vi "PCDeviceInit.vi"(10 "error in (no error)":errorcluster) -> ()   [LabVIEW 2011]
uses:
  Utilities/controls/ctlSeqFNs_Main.ctl
  Utilities/controls/ctlSeqFNs_AVTGuppy.ctl
  Utilities/controls/ctlSeqFNs_CTIOTF.ctl
  Utilities/controls/ctlSeqFNs_Koheras.ctl
  Utilities/controls/ctlSeqFNs_PCDeviceInit.ctl
  Utilities/controls/ctlSeqFNs_Scanner.ctl
  Utilities/controls/ctlSeqFNs_Andor.ctl
  <vilib>/userDefined/High Color/IMAQdx.ctl
panel:
  in  "config remote device":T2
  in  "initDevData":T3
  in  "StatusTerminal":string[](array[string])
  in  "remote device online status":T4
  in  "interface management remote device":T5
  in  "set remote device online":T4
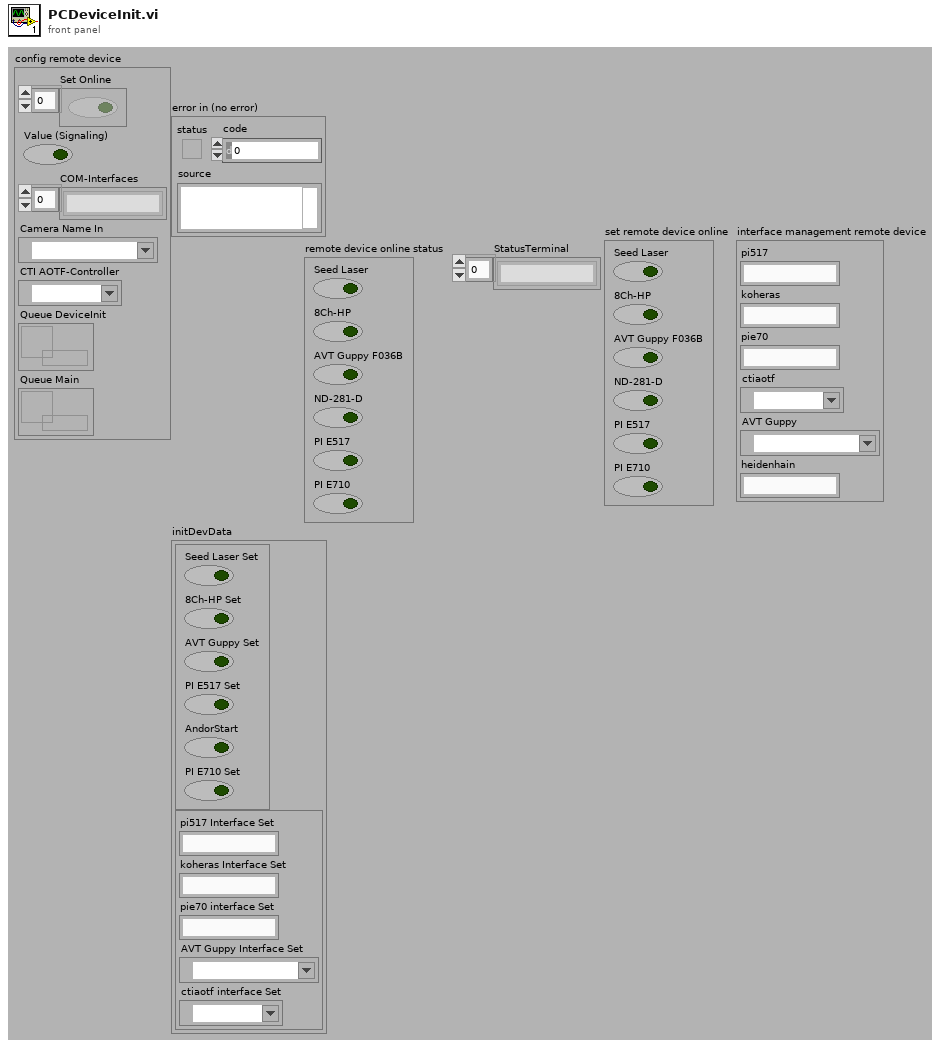
[diagram p1: front panel]
types:
  T1 = typedef "IMAQdx.ctl" = refnum<k21>
  T2 = cluster{"Set Online":bool[], "Value (Signaling)":bool, "COM-Interfaces":string[], "Camera Name In":T1, "CTI AOTF-Controller":refnum<visa-resource-name>, "Queue DeviceInit":refnum<queue>, "Queue Main":refnum<queue>}
  T3 = cluster{cluster{"Seed Laser Set":bool, "8Ch-HP Set":bool, "AVT Guppy Set":bool, "PI E517 Set":bool, "AndorStart":bool, "PI E710 Set":bool}, cluster{"pi517 Interface Set":string, "koheras Interface Set":string, "pie70 interface Set":string, "AVT Guppy Interface Set":T1, "ctiaotf interface Set":refnum<visa-resource-name>}}
  T4 = cluster{"Seed Laser":bool, "8Ch-HP":bool, "AVT Guppy F036B":bool, "ND-281-D":bool, "PI E517":bool, "PI E710":bool}
  T5 = cluster{"pi517":string, "koheras":string, "pie70":string, "ctiaotf":refnum<visa-resource-name>, "AVT Guppy":T1, "heidenhain":string}
  T6 = typedef "ctlSeqFNs_PCDeviceInit.ctl" = enum16{"ERROR", "INIT", "ErrorDevice", "StartDevice", "DeviceStatus", "StopDevice", "EXIT", "IDLE"}
  T7 = cluster{"Queue Main":refnum<queue>, "Queue Andor":refnum<queue>, "Queue Scanner":refnum<queue>, "Queue Koheras":refnum<queue>, "Queue CTIOTF":refnum<queue>, "Queue AVTGuppy":refnum<queue>, "set remote device online":cluster{"Seed Laser":bool, "8Ch-HP":bool, "AVT Guppy F036B":bool, "ND-281-D":bool, "PI E517":bool, "PI E710":bool}, "config remote device":cluster{"Set Online":bool[], "Value (Signaling)":bool, "COM-Interfaces":string[], "Camera Name In":T1, "CTI AOTF-Controller":refnum<visa-resource-name>, "Queue DeviceInit":refnum<queue>, "Queue Main":refnum<queue>}, "remote device online status":cluster{"Seed Laser":bool, "8Ch-HP":bool, "AVT Guppy F036B":bool, "ND-281-D":bool, "PI E517":bool, "PI E710":bool}, "interface management remote device":cluster{"pi517":string, "koheras":string, "pie70":string, "ctiaotf":refnum<visa-resource-name>, "AVT Guppy":T1, "heidenhain":string}, "StatusTerminal":string[], "initDevData":cluster{cluster{"Seed Laser Set":bool, "8Ch-HP Set":bool, "AVT Guppy Set":bool, "PI E517 Set":bool, "AndorStart":bool, "PI E710 Set":bool}, cluster{"pi517 Interface Set":string, "koheras Interface Set":string, "pie70 interface Set":string, "AVT Guppy Interface Set":T1, "ctiaotf interface Set":refnum<visa-resource-name>}}}
  T8 = typedef "ctlSeqFNs_Koheras.ctl" = enum16{"ERROR", "INIT", "Initialization", "Configuration", "Measurement", "Shutdown", "IDLE", "EXIT"}
  T9 = typedef "ctlSeqFNs_Andor.ctl" = enum16{"ERROR", "INIT", "Initialization", "Configuration", "Measurement", "Shutdown", "IDLE", "EXIT"}
  T10 = typedef "ctlSeqFNs_Scanner.ctl" = enum16{"ERROR", "INIT", "Initialization", "Configuration", "Measurement", "Shutdown", "IDLE", "EXIT"}
  T11 = typedef "ctlSeqFNs_CTIOTF.ctl" = enum16{"ERROR", "INIT", "Initialization", "Configuration", "Measurement", "Shutdown", "IDLE", "EXIT"}
  T12 = typedef "ctlSeqFNs_AVTGuppy.ctl" = enum16{"ERROR", "INIT", "Initialization", "Configuration", "Measurement", "Shutdown", "IDLE", "EXIT"}
  T13 = typedef "ctlSeqFNs_Main.ctl" = enum16{"ERROR", "INIT", "CONFIGURE", "MEASUREMENT", "SHUTDOWN", "IDLE", "EXIT"}
  T14 = cluster{"pi517 Interface Set":string, "pie70 interface Set":string, "PI E710":bool, "PI E517":bool}
  T15 = cluster{"Koheras":bool, "AOTF":bool, "ctiaotf interface Set":refnum<visa-resource-name>, "koheras Interface Set":string}
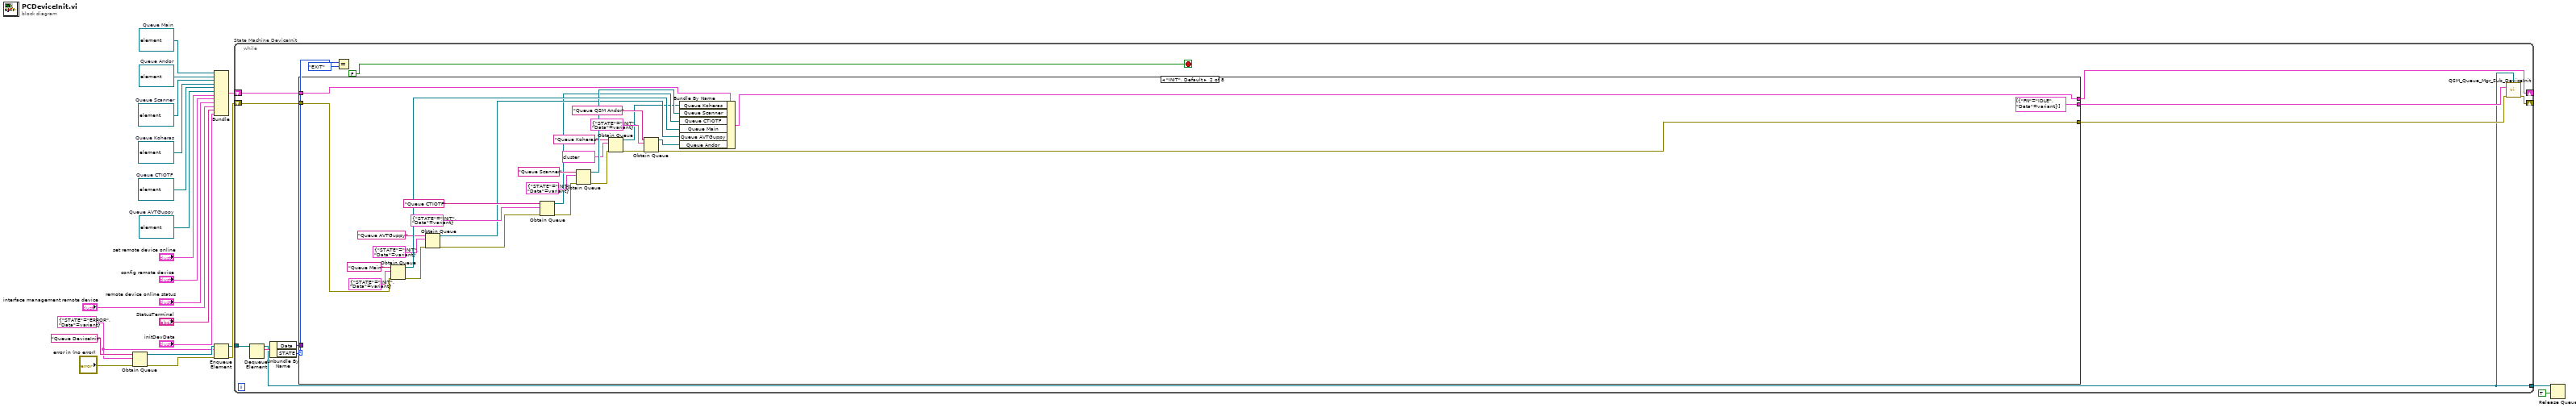
[diagram p0: block diagram]
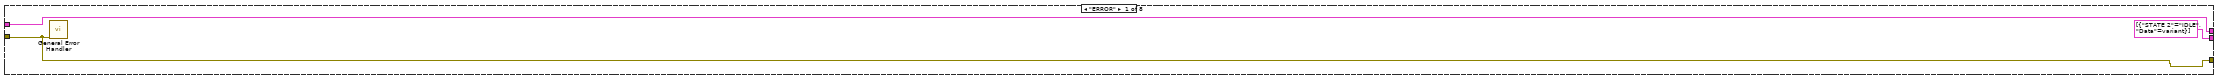
[diagram p2: hidden frame]
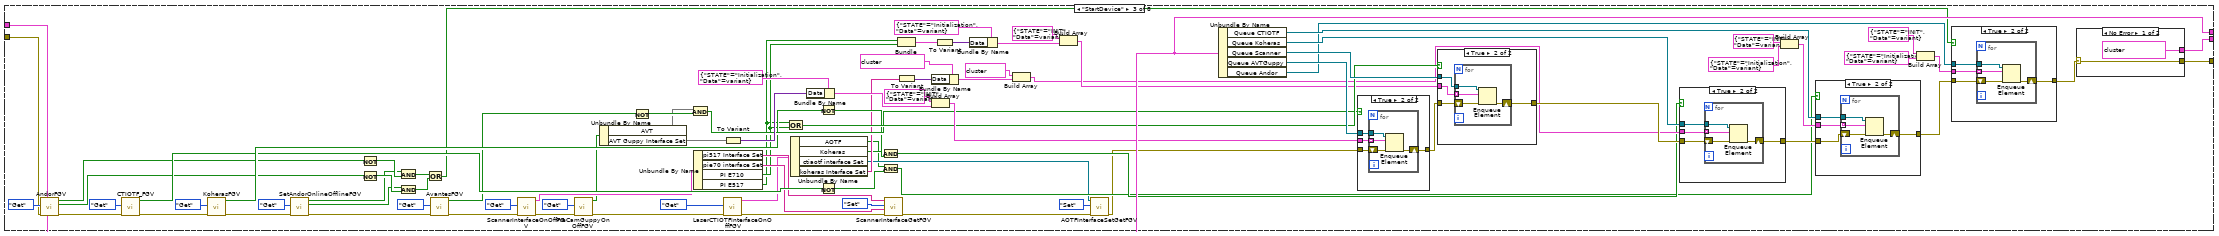
[diagram p3: hidden frame]
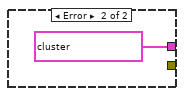
[diagram p9: hidden frame]
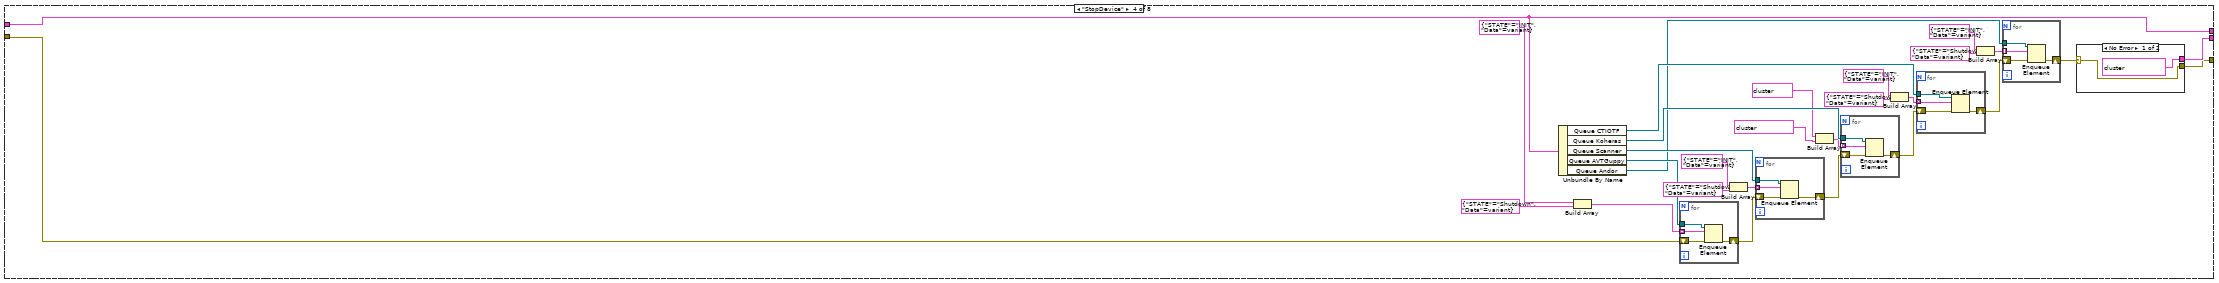
[diagram p10: hidden frame]
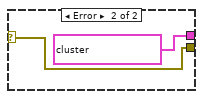
[diagram p11: hidden frame]
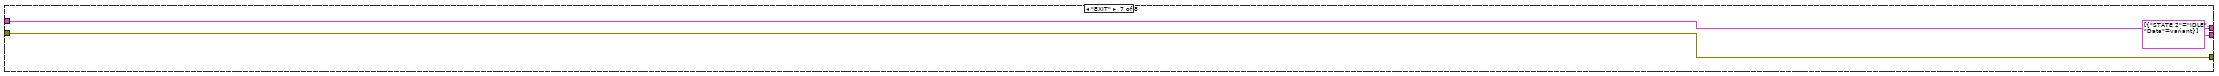
[diagram p14: hidden frame]
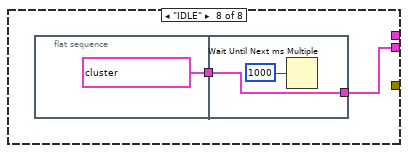
[diagram p15: hidden frame]
diagram:
  w1 = refnum<queue> refnum  # Queue Koheras
  w5 = refnum<queue> refnum  # Queue Andor
  w6 = refnum<queue> refnum  # Queue CTIOTF
  w7 = refnum<queue> refnum  # Queue AVTGuppy
  w9 = refnum<queue> refnum  # Queue Scanner
  w4 = refnum<queue> refnum  # Queue Main
  w14 = cluster{"STATE":T6, "Data":variant} {"STATE"=enum."ERROR", "Data"=variant} ("element")
  n1 = Obtain Queue(name (unnamed)="Queue DeviceInit", element data type=w14, error in (no error)="error in (no error)") -> (queue out=w19:refnum<queue>, error out=w21:errorcluster)  [unwired: 2 in, 1 out]
  n2 = Bundle("Queue Main"=w4, "Queue Andor"=w5, "Queue Scanner"=w9, "Queue Koheras"=w1, "Queue CTIOTF"=w6, "Queue AVTGuppy"=w7, "set remote device online"="set remote device online", "config remote device"="config remote device", "remote device online status"="remote device online status", "interface management remote device"="interface management remote device", "StatusTerminal"="StatusTerminal", "initDevData"="initDevData") -> (w18:T7)  [unwired: 1 in]
  n3 = Enqueue Element(queue=w19, element=w14, error in (no error)=w21) -> (queue out=w15:refnum<queue>, error out=w20:errorcluster)  [unwired: 1 in, 1 out]
  n4 = while "State Machine DeviceInit" {
    shift-right: [w28] -> _
    shift-left: w20 -> [w35]
    tunnel: w15 -> [w34]
    tunnel: [w26] -> w17
    shift-right: [w30] -> _
    shift-left: w18 -> [w31]
    stop <- FALSE ("x = y?") stop-if-true
    n5 = Dequeue Element(queue=w34) -> (queue out=w26:refnum<queue>, element=w33:cluster{"STATE":T6, "Data":variant})  [unwired: 2 in, 2 out]
    n6 = Unbundle By Name(w33) -> ("Data"=w32:variant, "STATE"=w25:T6)
    n7 = case shown="\"INIT\", Default" w25 {
      tunnel: w35 -> [w36 w65 w91 w205 w256 _ w260 _]
      tunnel: w32 -> [_ _ _ _ _ _ _ _]
      tunnel: w31 -> [w38 w66 w154 w206 w257 _ w259 _]
      tunnel: [w38 w48 w154 w206 w257 _ w259 _] -> w30
      tunnel: [cluster{"STATE 2":T6, "Data":variant}[] [{"STATE 2"=enum."IDLE", "Data"=variant}] cluster{"FN":T6, "Data":variant}[] [{"FN"=enum."IDLE", "Data"=variant}] w150 w231 _ _ cluster{"STATE 2":T6, "Data":variant}[] [{"STATE 2"=enum."IDLE", "Data"=variant}] w261] -> w27
      tunnel: [w36 w44 w149 w230 w256 _ w260 _] -> w29
      frame "ERROR" {
        n8 = call <vilib>:"General Error Handler.vi"("error in (no error)"=w36) -> ()  [unwired: 10 in, 5 out]
      }
      frame "INIT", Default {
        n9 = Obtain Queue(name (unnamed)="Queue Main" ("Queue Name"), element data type=cluster{"STATE":T13, "Data":variant} {"STATE"=enum."INIT", "Data"=variant} ("element"), error in (no error)=w65) -> (queue out=w62:refnum<queue>, error out=w60:errorcluster)  [unwired: 2 in, 1 out]
        n10 = Obtain Queue(name (unnamed)="Queue AVTGuppy" ("Queue Name"), element data type=cluster{"STATE":T12, "Data":variant} {"STATE"=enum."INIT", "Data"=variant} ("element"), error in (no error)=w60) -> (queue out=w51:refnum<queue>, error out=w55:errorcluster)  [unwired: 2 in, 1 out]
        n11 = Obtain Queue(name (unnamed)="Queue CTIOTF", element data type=cluster{"STATE":T11, "Data":variant} {"STATE"=enum."INIT", "Data"=variant} ("element"), error in (no error)=w55) -> (queue out=w47:refnum<queue>, error out=w52:errorcluster)  [unwired: 2 in, 1 out]
        n12 = Obtain Queue(name (unnamed)="Queue Scanner", element data type=cluster{"STATE":T10, "Data":variant} {"STATE"=enum."INIT", "Data"=variant} ("element"), error in (no error)=w52) -> (queue out=w54:refnum<queue>, error out=w53:errorcluster)  [unwired: 2 in, 1 out]
        n13 = Obtain Queue(name (unnamed)="Queue Koheras", element data type=cluster{"Data":variant, "FGV_Control":T8} {"Data"=variant, "FGV_Control"=enum."INIT"} ("element"), error in (no error)=w53) -> (queue out=w39:refnum<queue>, error out=w45:errorcluster)  [unwired: 2 in, 1 out]
        n14 = Obtain Queue(name (unnamed)="Queue QSM Andor", element data type=cluster{"STATE":T9, "Data":variant} {"STATE"=enum."INIT", "Data"=variant} ("element"), error in (no error)=w45) -> (queue out=w43:refnum<queue>, error out=w44:errorcluster)  [unwired: 2 in, 1 out]
        n15 = Bundle By Name(cluster=w66, "Queue Koheras"=w39, "Queue Scanner"=w54, "Queue CTIOTF"=w47, "Queue Main"=w62, "Queue AVTGuppy"=w51, "Queue Andor"=w43) -> (w48:T7)
      }
      frame "StartDevice" {
        n16 = call "AndorFGV.vi"("error in"=w91, "Set_Get"=enum16{"Set", "Get"}."Get") -> ("error out"=w90:errorcluster, "andor 1"=w100:bool, "andor 0"=w110:bool)  [unwired: 7 in]
        n17 = call "CTIOTF_FGV.vi"("error in"=w90, "Set_Get"=enum16{"Set", "Get"}."Get") -> ("error out"=w89:errorcluster, "aotfGet"=w112:bool)  [unwired: 8 in]
        n18 = call "KoherasFGV.vi"("error in"=w89, "Set_Get"=enum16{"Set", "Get"}."Get") -> ("error out"=w71:errorcluster, "Get"=w114:bool)  [unwired: 8 in]
        n19 = call "SetAndorOnlineOfflineFGV.vi"("error in"=w71, "Set_Get"=enum16{"Set", "Get"}."Get") -> ("error out"=w70:errorcluster, "andor 1"=w67:bool, "andor 0"=w68:bool)  [unwired: 7 in]
        n20 = Not(x=w110) -> (.not. x?=w109:bool)
        n21 = Not(x=w100) -> (.not. x?=w101:bool)
        n22 = And(x=w68, y=w109) -> (x .and. y?=w98:bool)
        n23 = And(x=w67, y=w101) -> (x .and. y?=w97:bool)
        n24 = Or(x=w98, y=w97) -> (x .or. y?=w99:bool)
        n25 = call "AvantesFGV.vi"("error in"=w70, "Set_Get"=enum16{"Set", "Get"}."Get") -> ("error out"=w88:errorcluster, "Get"=w108:bool)  [unwired: 8 in]
        n26 = call "ScannerInterfaceOnOffFGV.vi"("error in"=w88, "Set_Get"=enum16{"Set", "Get"}."Get") -> ("error out"=w94:errorcluster, "ScannerInterfaceOUT"=w84:T14)  [unwired: 8 in]
        n27 = call "PreCamGuppyOnOffFGV.vi"("error in"=w94, "Set_Get"=enum16{"Set", "Get"}."Get") -> ("error out"=w93:errorcluster, "out"=w79:bool)  [unwired: 8 in]
        n28 = Unbundle By Name(w79) -> ("AVT"=w77, "AVT Guppy Interface Set"=w78)
        n29 = Not(x=w108) -> (.not. x?=w107:bool)
        n30 = And(x=w77, y=w107) -> (x .and. y?=w120:bool)
        n31 = Unbundle By Name(w84) -> ("pi517 Interface Set"=w83:string, "pie70 interface Set"=w82:string, "PI E710"=w81:bool, "PI E517"=w80:bool)
        n32 = call "LaserCTIOTFInterfaceOnOffFGV.vi"("error in"=w93, "Set_Get"=enum16{"Set", "Get"}."Get") -> ("error out"=w92:errorcluster, "LaserCtiotfInterfaceOnOffOUT"=w76:T15)  [unwired: 8 in]
        n33 = To Variant(anything=w78) -> (Variant=w152:variant)
        n34 = Or(x=w80, y=w81) -> (x .or. y?=w142:bool)
        n35 = Unbundle By Name(w76) -> ("AOTF"=w72:bool, "Koheras"=w73:bool, "ctiaotf interface Set"=w74:refnum<visa-resource-name>, "koheras Interface Set"=w75:string)
        n36 = Bundle By Name(cluster=cluster{"STATE":T12, "Data":variant} {"STATE"=enum."Initialization", "Data"=variant} ("element"), "Data"=w152) -> (w148:cluster{"STATE":T12, "Data":variant})
        n37 = Not(x=w114) -> (.not. x?=w113:bool)
        n38 = Not(x=w112) -> (.not. x?=w111:bool)
        n39 = And(x=w73, y=w113) -> (x .and. y?=w124:bool)
        n40 = And(x=w72, y=w111) -> (x .and. y?=w122:bool)
        n41 = call "ScannerInterfaceGetFGV.vi"("error in"=w92, "pie70 interface Set"=w82, "FGV_Control"=enum16{"Set", "Get"}."Set", "pi517 Interface Set"=w83) -> ("error out"=w103:errorcluster)  [unwired: 5 in, 2 out]
        n42 = Bundle("PI E517"=w80, "PI E710"=w81) -> (w115:cluster{"PI E517":bool, "PI E710":bool})  [unwired: 1 in]
        n43 = To Variant(anything=w75) -> (Variant=w151:variant)
        n44 = Bundle By Name(cluster=cluster{"Data":variant, "FGV_Control":T8} {"Data"=variant, "FGV_Control"=enum."Initialization"} ("element"), "Data"=w151) -> (w137:cluster{"Data":variant, "FGV_Control":T8})
        n45 = Build Array(cluster{"STATE":T12, "Data":variant} {"STATE"=enum."INIT", "Data"=variant} ("element"), w148) -> (w146:cluster{"STATE":T12, "Data":variant}[])
        n46 = To Variant(anything=w115) -> (Variant=w116:variant)
        n47 = Bundle By Name(cluster=cluster{"STATE":T10, "Data":variant} {"STATE"=enum."Initialization", "Data"=variant} ("element"), "Data"=w116) -> (w117:cluster{"STATE":T10, "Data":variant})
        n48 = Build Array(cluster{"Data":variant, "FGV_Control":T8} {"Data"=variant, "FGV_Control"=enum."INIT"} ("element"), w137) -> (w136:cluster{"Data":variant, "FGV_Control":T8}[])
        n49 = Build Array(cluster{"STATE":T10, "Data":variant} {"STATE"=enum."INIT", "Data"=variant} ("element"), w117) -> (w141:cluster{"STATE":T10, "Data":variant}[])
        n50 = call "AOTFInterfaceSetGetFGV.vi"("error in"=w103, "FGV_Control"=enum16{"Set", "Get"}."Set", "ctiaotf interface Set"=w74) -> ("error out"=w102:errorcluster)  [unwired: 7 in, 1 out]
        n51 = Unbundle By Name(w154) -> ("Queue CTIOTF"=w135:refnum<queue>, "Queue Koheras"=w138:refnum<queue>, "Queue Scanner"=w143:refnum<queue>, "Queue AVTGuppy"=w145:refnum<queue>, "Queue Andor"=w131:refnum<queue>)
        n52 = case shown="True" w120 {
          tunnel: [w191 w195] -> w144
          tunnel: w102 -> [w191 w194]
          tunnel: w146 -> [_ w193]
          tunnel: w145 -> [_ w192]
          frame False {
          }
          frame True {
            n53 = for {
              tunnel: w192 -> [w199]
              shift-right: [w197] -> w195
              shift-left: w194 -> [w198]
              tunnel: w193 -> [w196] mode=indexing
              n54 = Enqueue Element(queue=w199, element=w196, error in (no error)=w198) -> (error out=w197:errorcluster)  [unwired: 1 in, 2 out]
            }
          }
        }
        n55 = case shown="True" w142 {
          tunnel: [w182 w186] -> w139
          tunnel: w144 -> [w182 w185]
          tunnel: w141 -> [_ w184]
          tunnel: w143 -> [_ w183]
          frame False {
          }
          frame True {
            n56 = for {
              tunnel: w183 -> [w190]
              shift-right: [w188] -> w186
              shift-left: w185 -> [w189]
              tunnel: w184 -> [w187] mode=indexing
              n57 = Enqueue Element(queue=w190, element=w187, error in (no error)=w189) -> (error out=w188:errorcluster)  [unwired: 1 in, 2 out]
            }
          }
        }
        n58 = case shown="True" w124 {
          tunnel: [w173 w177] -> w132
          tunnel: w139 -> [w173 w176]
          tunnel: w136 -> [_ w175]
          tunnel: w138 -> [_ w174]
          frame False {
          }
          frame True {
            n59 = for {
              tunnel: w174 -> [w181]
              shift-right: [w179] -> w177
              shift-left: w176 -> [w180]
              tunnel: w175 -> [w178] mode=indexing
              n60 = Enqueue Element(queue=w181, element=w178, error in (no error)=w180) -> (error out=w179:errorcluster)  [unwired: 1 in, 2 out]
            }
          }
        }
        n61 = Build Array(cluster{"STATE":T11, "Data":variant} {"STATE"=enum."INIT", "Data"=variant} ("element"), cluster{"STATE":T11, "Data":variant} {"STATE"=enum."Initialization", "Data"=variant} ("element")) -> (w133:cluster{"STATE":T11, "Data":variant}[])
        n62 = case shown="True" w122 {
          tunnel: [w164 w168] -> w130
          tunnel: w132 -> [w164 w167]
          tunnel: w133 -> [_ w166]
          tunnel: w135 -> [_ w165]
          frame False {
          }
          frame True {
            n63 = for {
              tunnel: w165 -> [w172]
              shift-right: [w170] -> w168
              shift-left: w167 -> [w171]
              tunnel: w166 -> [w169] mode=indexing
              n64 = Enqueue Element(queue=w172, element=w169, error in (no error)=w171) -> (error out=w170:errorcluster)  [unwired: 1 in, 2 out]
            }
          }
        }
        n65 = Build Array(cluster{"STATE":T9, "Data":variant} {"STATE"=enum."INIT", "Data"=variant} ("element"), cluster{"STATE":T9, "Data":variant} {"STATE"=enum."Initialization", "Data"=variant} ("element")) -> (w126:cluster{"STATE":T9, "Data":variant}[])
        n66 = case shown="True" w99 {
          tunnel: [w155 w159] -> w129
          tunnel: w130 -> [w155 w158]
          tunnel: w126 -> [_ w157]
          tunnel: w131 -> [_ w156]
          frame False {
          }
          frame True {
            n67 = for {
              tunnel: w156 -> [w163]
              shift-right: [w161] -> w159
              shift-left: w158 -> [w162]
              tunnel: w157 -> [w160] mode=indexing
              n68 = Enqueue Element(queue=w163, element=w160, error in (no error)=w162) -> (error out=w161:errorcluster)  [unwired: 1 in, 2 out]
            }
          }
        }
        n69 = case shown="No Error" w129 {
          selector: w129 -> [w201 _]
          tunnel: [w201 _] -> w149
          tunnel: [cluster{"STATE 2":T6, "Data":variant}[] [{"STATE 2"=enum."IDLE", "Data"=variant}, {"STATE 2"=enum."StopDevice", "Data"=variant}, {"STATE 2"=enum."EXIT", "Data"=variant}, {"STATE 2"=enum."IDLE", "Data"=variant}, {"STATE 2"=enum."DeviceStatus", "Data"=variant}] cluster{"STATE 2":T6, "Data":variant}[] [{"STATE 2"=enum."IDLE", "Data"=variant}, {"STATE 2"=enum."StopDevice", "Data"=variant}, {"STATE 2"=enum."EXIT", "Data"=variant}, {"STATE 2"=enum."IDLE", "Data"=variant}, {"STATE 2"=enum."DeviceStatus", "Data"=variant}]] -> w150
          frame No Error {
          }
          frame Error {
          }
        }
      }
      frame "StopDevice" {
        n70 = Unbundle By Name(w206) -> ("Queue CTIOTF"=w219:refnum<queue>, "Queue Koheras"=w221:refnum<queue>, "Queue Scanner"=w225:refnum<queue>, "Queue AVTGuppy"=w227:refnum<queue>, "Queue Andor"=w216:refnum<queue>)
        n71 = Build Array(cluster{"STATE":T12, "Data":variant} {"STATE"=enum."INIT", "Data"=variant} ("element"), cluster{"STATE":T12, "Data":variant} {"STATE"=enum."Shutdown", "Data"=variant} ("element")) -> (w228:cluster{"STATE":T12, "Data":variant}[])
        n72 = for {
          tunnel: w227 -> [w251]
          shift-right: [w249] -> w226
          shift-left: w205 -> [w250]
          tunnel: w228 -> [w248] mode=indexing
          n73 = Enqueue Element(queue=w251, element=w248, error in (no error)=w250) -> (error out=w249:errorcluster)  [unwired: 1 in, 2 out]
        }
        n74 = Build Array(cluster{"STATE":T10, "Data":variant} {"STATE"=enum."INIT", "Data"=variant} ("element"), cluster{"STATE":T10, "Data":variant} {"STATE"=enum."Shutdown", "Data"=variant} ("element")) -> (w224:cluster{"STATE":T10, "Data":variant}[])
        n75 = for {
          tunnel: w225 -> [w247]
          shift-right: [w245] -> w222
          shift-left: w226 -> [w246]
          tunnel: w224 -> [w244] mode=indexing
          n76 = Enqueue Element(queue=w247, element=w244, error in (no error)=w246) -> (error out=w245:errorcluster)  [unwired: 1 in, 2 out]
        }
        n77 = Build Array(cluster{"Data":variant, "FGV_Control":T8} {"Data"=variant, "FGV_Control"=enum."INIT"} ("element"), cluster{"Data":variant, "FGV_Control":T8} {"Data"=variant, "FGV_Control"=enum."Shutdown"} ("element")) -> (w220:cluster{"Data":variant, "FGV_Control":T8}[])
        n78 = for {
          tunnel: w221 -> [w243]
          shift-right: [w241] -> w217
          shift-left: w222 -> [w242]
          tunnel: w220 -> [w240] mode=indexing
          n79 = Enqueue Element(queue=w243, element=w240, error in (no error)=w242) -> (error out=w241:errorcluster)  [unwired: 1 in, 2 out]
        }
        n80 = Build Array(cluster{"STATE":T11, "Data":variant} {"STATE"=enum."INIT", "Data"=variant} ("element"), cluster{"STATE":T11, "Data":variant} {"STATE"=enum."Shutdown", "Data"=variant} ("element")) -> (w218:cluster{"STATE":T11, "Data":variant}[])
        n81 = for {
          tunnel: w219 -> [w239]
          shift-right: [w237] -> w215
          shift-left: w217 -> [w238]
          tunnel: w218 -> [w236] mode=indexing
          n82 = Enqueue Element(queue=w239, element=w236, error in (no error)=w238) -> (error out=w237:errorcluster)  [unwired: 1 in, 2 out]
        }
        n83 = Build Array(cluster{"STATE":T9, "Data":variant} {"STATE"=enum."INIT", "Data"=variant} ("element"), cluster{"STATE":T9, "Data":variant} {"STATE"=enum."Shutdown", "Data"=variant} ("element")) -> (w211:cluster{"STATE":T9, "Data":variant}[])
        n84 = for {
          tunnel: w216 -> [w235]
          shift-right: [w233] -> w214
          shift-left: w215 -> [w234]
          tunnel: w211 -> [w232] mode=indexing
          n85 = Enqueue Element(queue=w235, element=w232, error in (no error)=w234) -> (error out=w233:errorcluster)  [unwired: 1 in, 2 out]
        }
        n86 = case shown="No Error" w214 {
          selector: w214 -> [w253 w255]
          tunnel: [w253 w255] -> w230
          tunnel: [cluster{"STATE 2":T6, "Data":variant}[] [{"STATE 2"=enum."IDLE", "Data"=variant}, {"STATE 2"=enum."IDLE", "Data"=variant}, {"STATE 2"=enum."EXIT", "Data"=variant}, {"STATE 2"=enum."IDLE", "Data"=variant}, {"STATE 2"=enum."DeviceStatus", "Data"=variant}] cluster{"STATE 2":T6, "Data":variant}[] [{"STATE 2"=enum."ERROR", "Data"=variant}, {"STATE 2"=enum."ERROR", "Data"=variant}, {"STATE 2"=enum."EXIT", "Data"=variant}, {"STATE 2"=enum."IDLE", "Data"=variant}, {"STATE 2"=enum."DeviceStatus", "Data"=variant}]] -> w231
          frame No Error {
          }
          frame Error {
          }
        }
      }
      frame "ErrorDevice" {
      }
      frame "DeviceStatus" {
      }
      frame "EXIT" {
      }
      frame "IDLE" {
        n87 = flat-sequence {
          tunnel: [cluster{"STATE 2":T6, "Data":variant}[] [{"STATE 2"=enum."IDLE", "Data"=variant}, {"STATE 2"=enum."IDLE", "Data"=variant}, {"STATE 2"=enum."EXIT", "Data"=variant}, {"STATE 2"=enum."IDLE", "Data"=variant}, {"STATE 2"=enum."DeviceStatus", "Data"=variant}]] -> w262
          tunnel: [w264] -> w261
          tunnel: w262 -> [w264]
          frame #0 {
          }
          frame #1 {
            n88 = Wait Until Next ms Multiple(millisecond multiple=u32 1000) -> ()  [unwired: 1 out]
          }
        }
      }
    }
    n89 = Equal?(x=w25, y=ctlSeqFNs_PCDeviceInit."EXIT") -> ()  [unwired: 1 out]
    n90 = call "QSM_Queue_Mgr_Sub_DeviceInit.vi"("queue out"=w26, "QSTATES"=w27, "Error IN"=w29) -> ("Error OUT"=w28:errorcluster)  [unwired: 12 in]
  }
  n91 = Release Queue(queue=w17, force destroy? (F)=TRUE) -> ()  [unwired: 1 in, 3 out]
